vi "EnFlo_Tun_Heater_Control.vi"(1 "Heaters Enabled time (s)":dbl, 2 "Heaters Just Enabled":bool, 3 "Ch Names":string[](array[string]), 4 "Values":dbl[](array[numeric]) format="%.2f") -> ()   [LabVIEW 2016]
uses:
  ADAM Client/Sub VIs/ADAM Controls/Search_mode.ctl
  <vilib>/Analysis/baseanly.llb/Mean (DBL).vi
  ADAM_Global.vi
  <vilib>/Analysis/NI_AALBase.lvlib
  <vilib>/Analysis/NI_AALPro.lvlib
panel:
  out "Upper limit on Power":dbl
  in  "Proportional Error Deadband":dbl=0.03
  out "Read Values OK":bool
  out "History Out":dbl[](array[numeric])
  out "Current Temp":dbl
  out "Setpoint":dbl
  out "Error Range":dbl
  in  "Index To Display":i32
  out "Feedback Temperature":string
  in  "Minimum Power Change in %":dbl=0.08
  in  "Total History":i32=450
  out "Proportional Term":dbl format="%#.1f"
  out "Control Sum":dbl format="%#.1f"
  out "Differential Term":dbl format="%#.1f"
  in  "Derivative History":i32=60
  out "Integral Term":dbl format="%#.1f"
  # "This is the Max - Min error for the Total History"
  # "When running at\nSteady Cond"
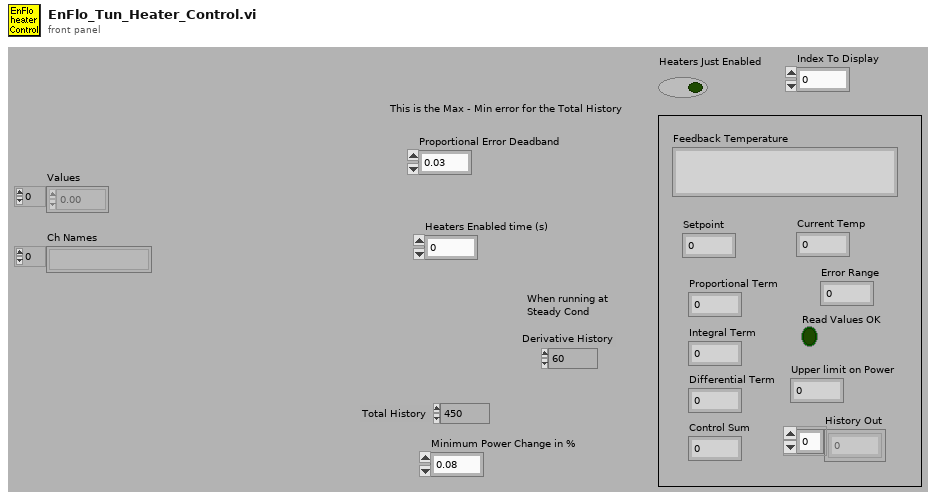
[diagram p1: front panel]
types:
  T1 = enum16{"On", "Off", "Always On", "Always Off", "Delete"}
  T2 = typedef "Search_mode.ctl" = enum16{"Between times", "All Times"}
  T3 = typedef "Ch_description_ADAM.ctl" = cluster{"Ch Name":string, "Type":T4, "Function":T5, "Ch State":T6, "Calibration type":T7, "A":dbl, "B":dbl, "C":dbl, "D":dbl, "Comments":string, "Address":T8, "String":string, "Duty":u16}
  T4 = typedef "Module_type_ADAM.ctl" = string
  T5 = typedef "Function_ADAM.ctl" = enum16{"Analogue Input", "Digital Input", "Event counter", "Event rate", "Analogue Output", "Digital Output", "Relay Output"}
  T6 = typedef "Channel_State.ctl" = enum16{"On", "Off", "Always On", "Always Off"}
  T7 = typedef "Calib_type_ADAM.ctl" = enum16{"Raw", "Bx + A", "Cx^2 + Bx + A", "Dx^3 + Cx^2 + Bx + A", "In Band", "Hi-Tec Q", "Hi-Tec M_dot", "Text"}
  T8 = typedef "Address.ctl" = cluster{"Main":i32, "Ch.":i32, "Sub":i32, "Port Name":string}
  T9 = cluster{"Centre Times":dbl[], "Output array":dbl[]}
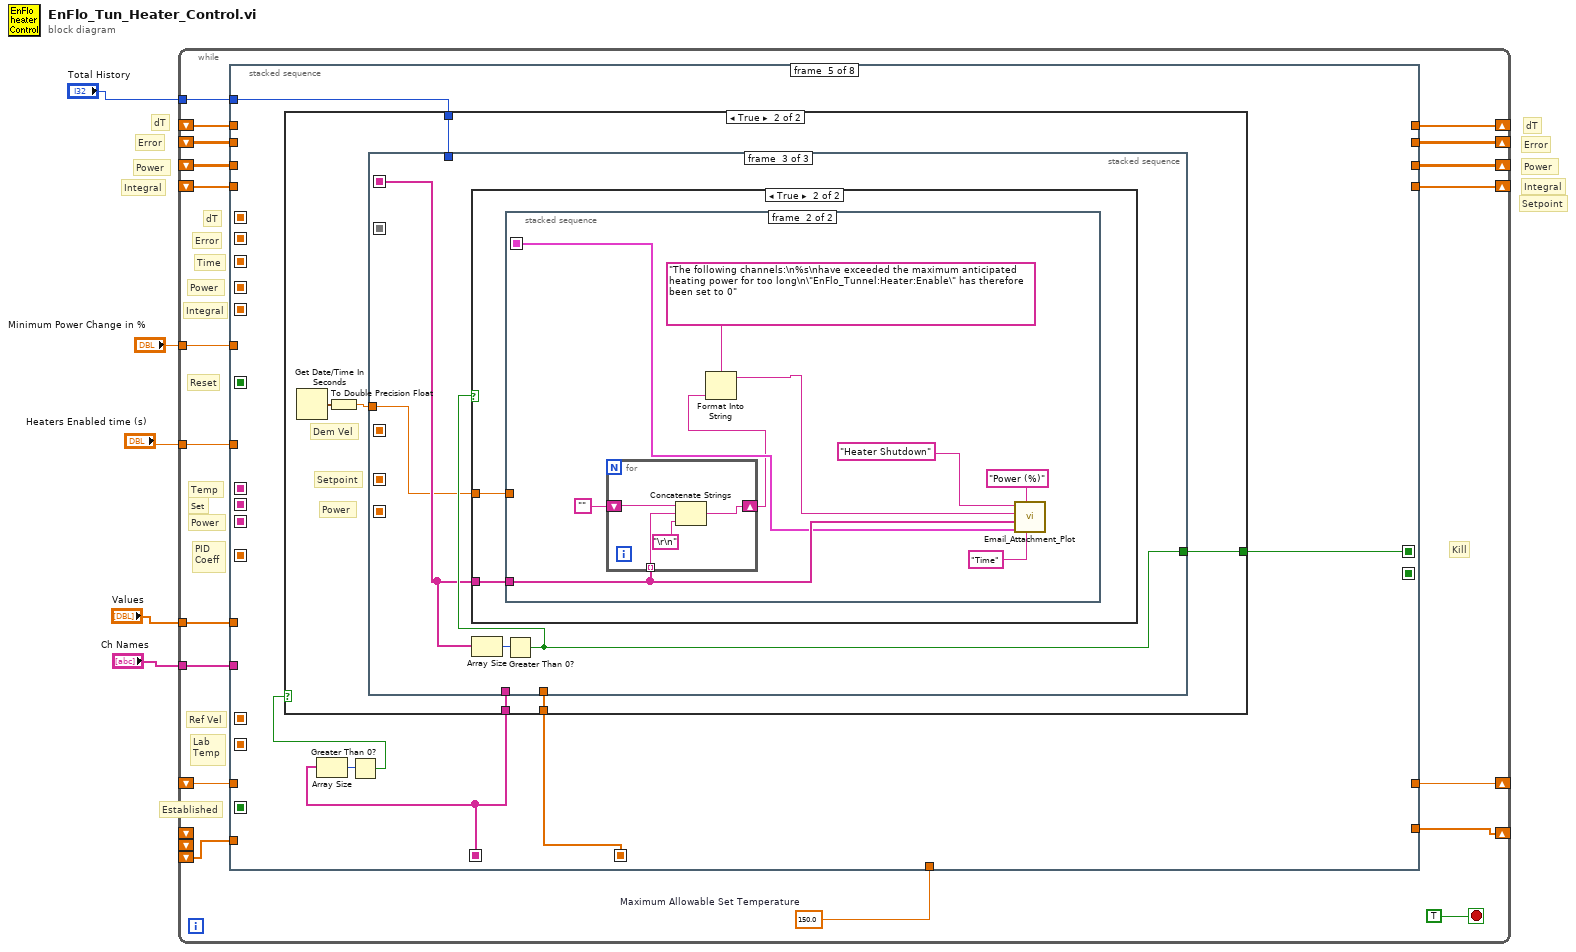
[diagram p0: block diagram]
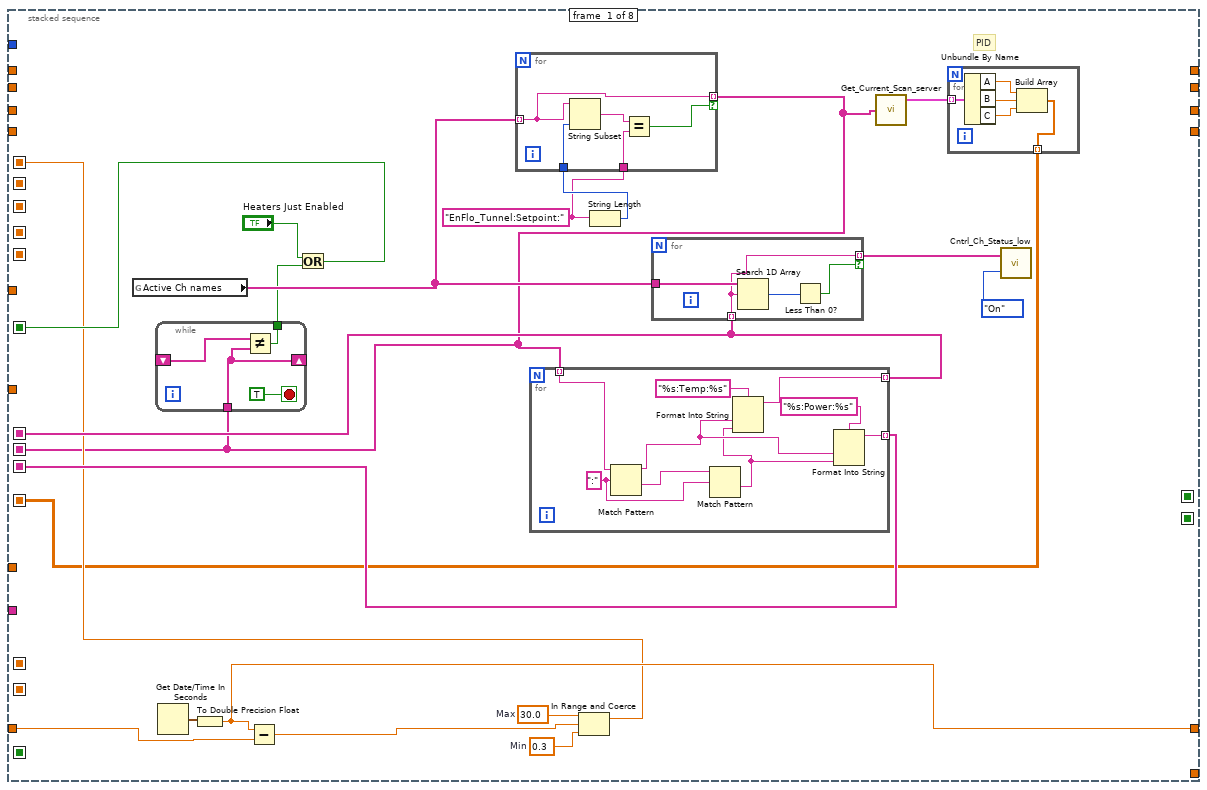
[diagram p2: hidden frame]
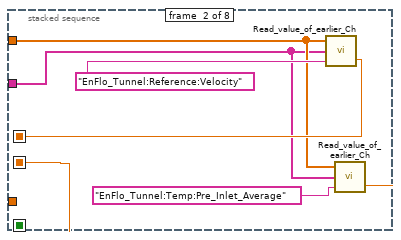
[diagram p3: hidden frame]
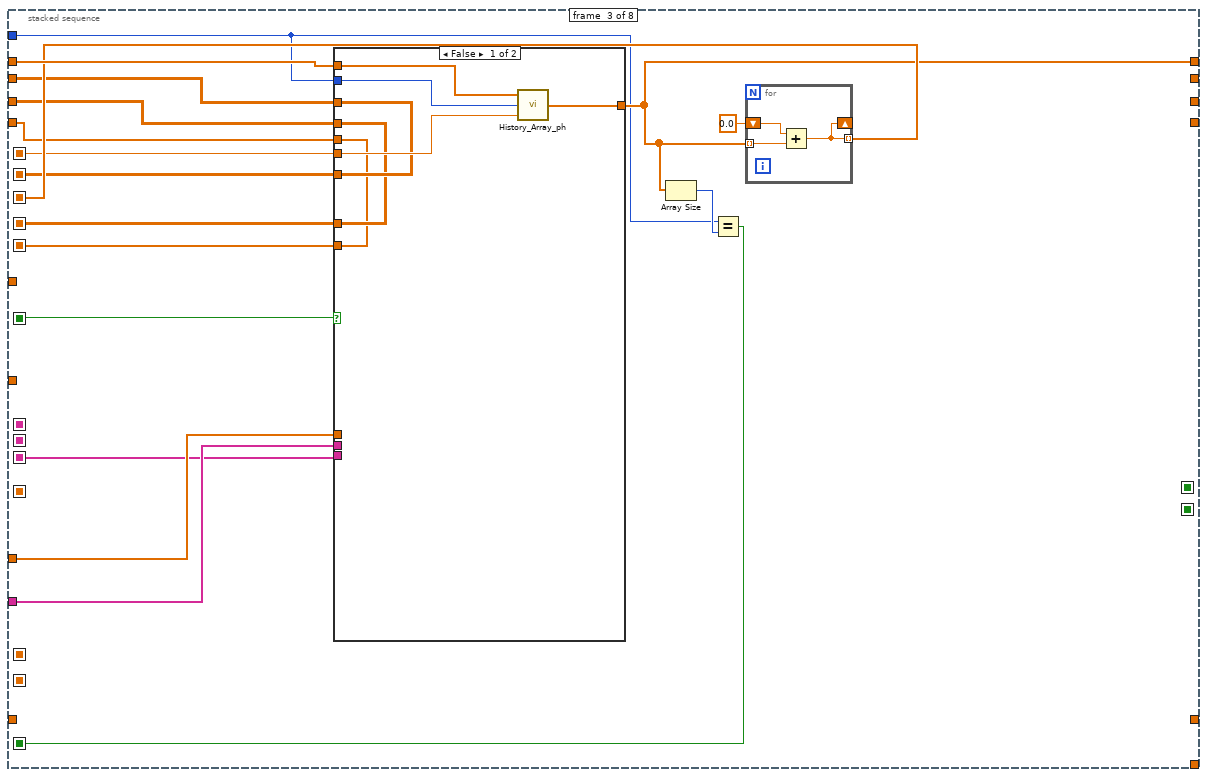
[diagram p4: hidden frame]
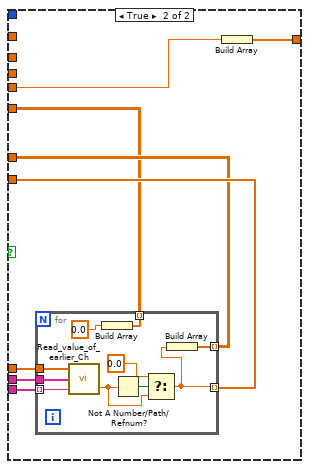
[diagram p5: hidden frame]
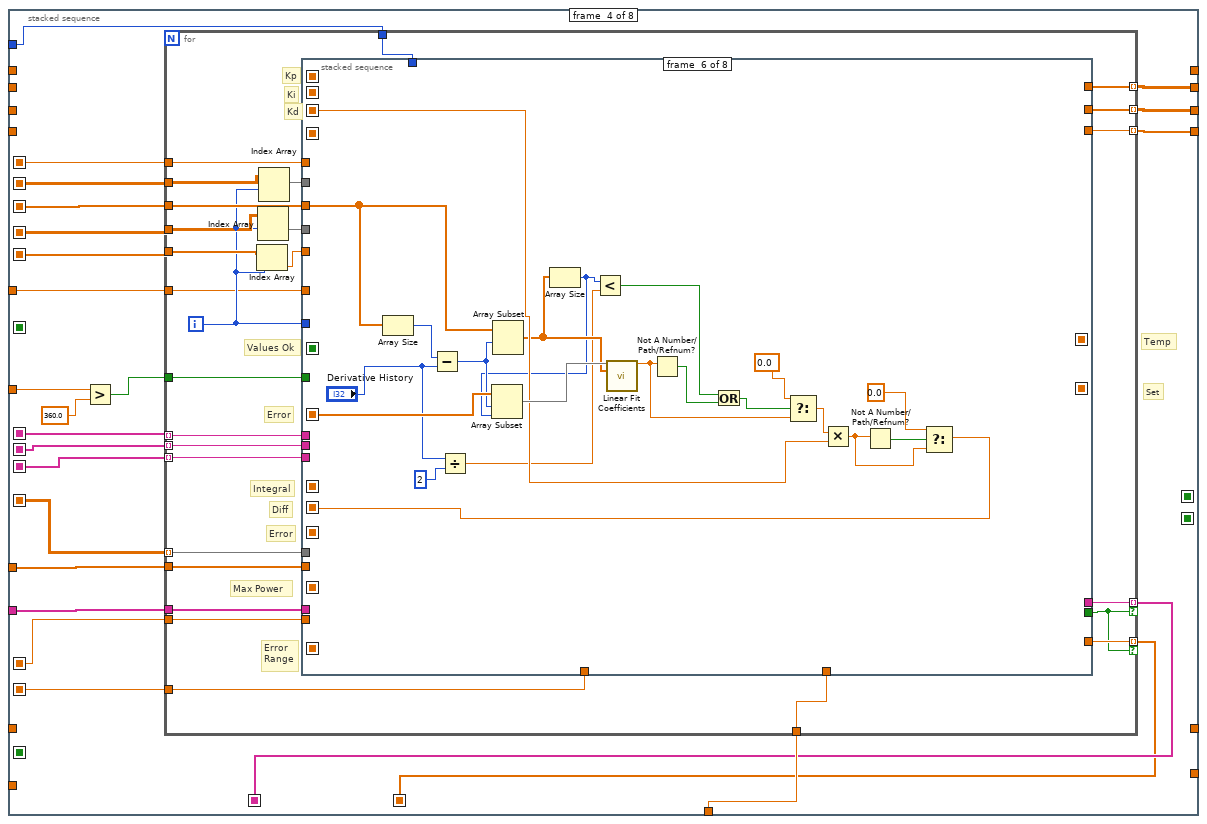
[diagram p6: hidden frame]
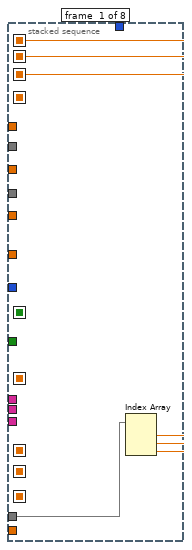
[diagram p7: hidden frame]
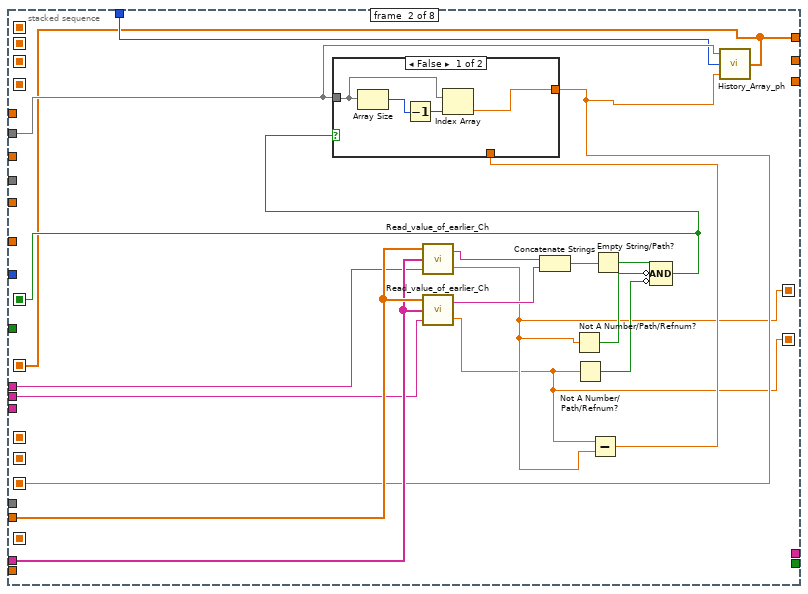
[diagram p8: hidden frame]
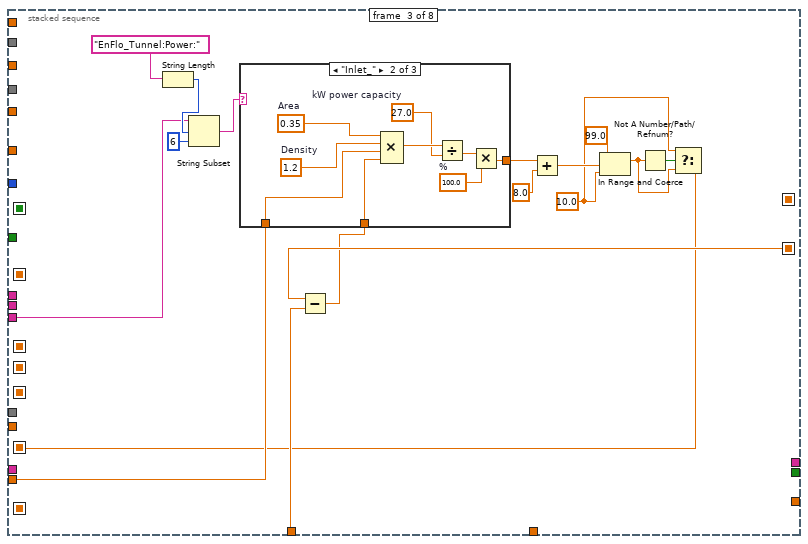
[diagram p10: hidden frame]
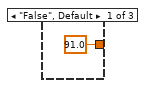
[diagram p11: hidden frame]
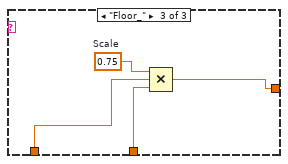
[diagram p12: hidden frame]
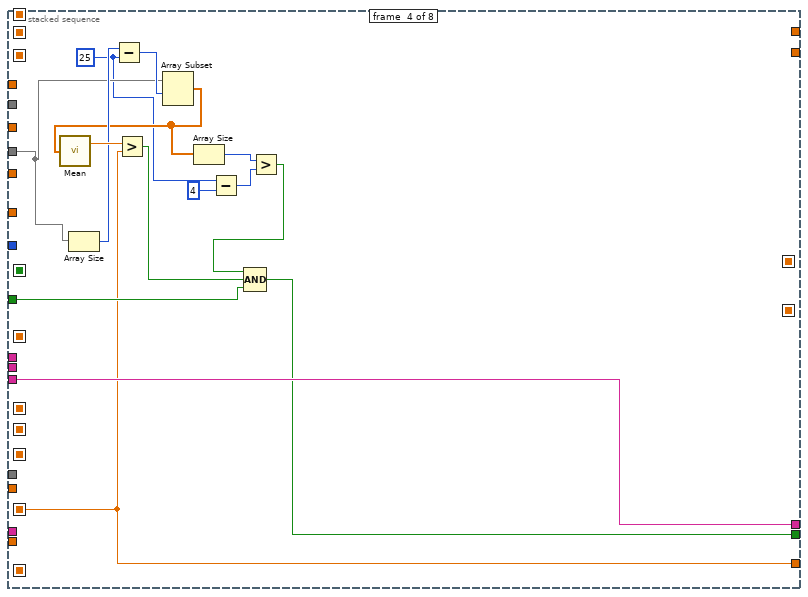
[diagram p13: hidden frame]
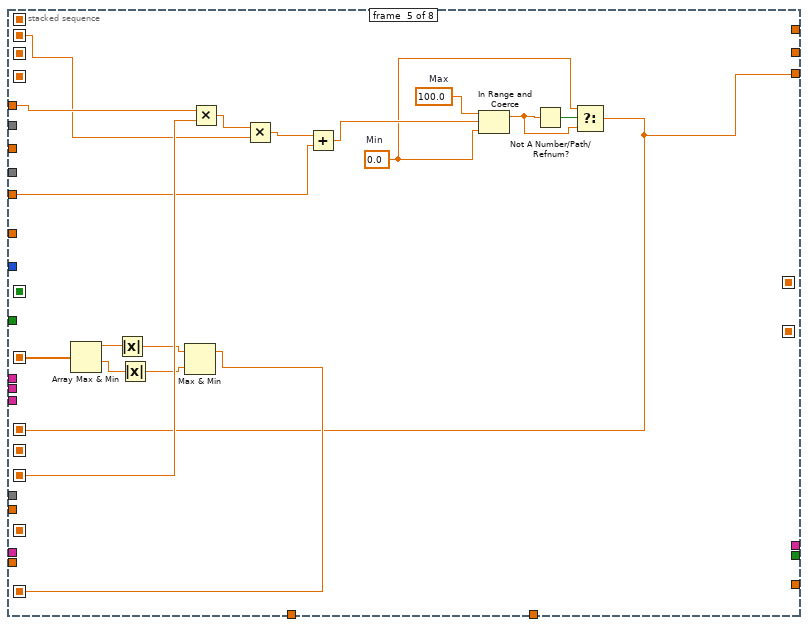
[diagram p14: hidden frame]
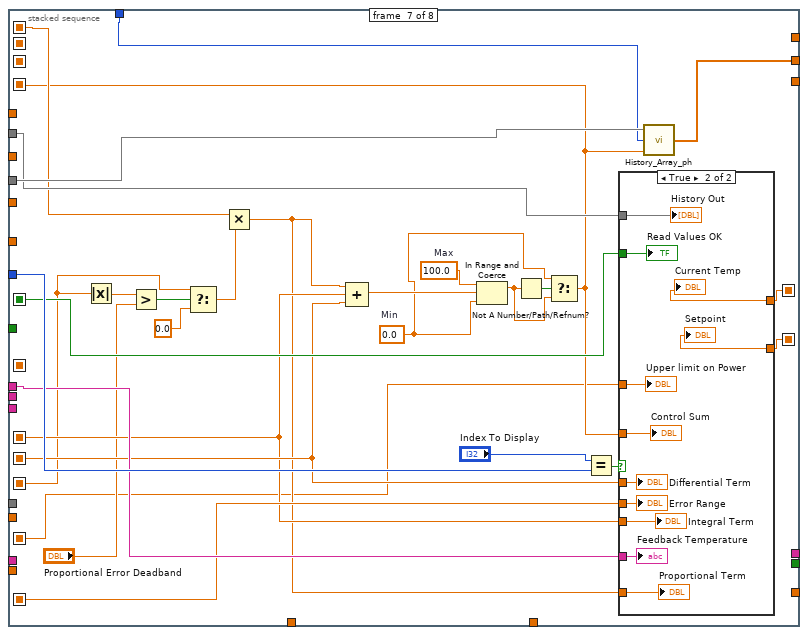
[diagram p15: hidden frame]
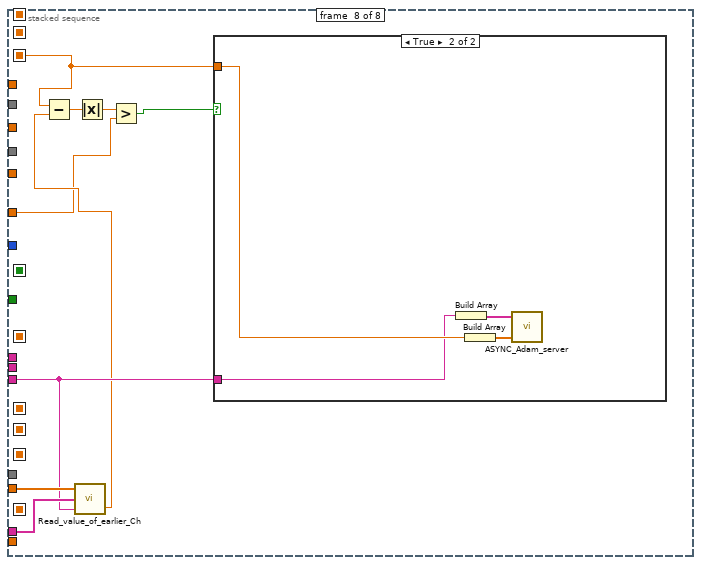
[diagram p17: hidden frame]
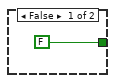
[diagram p19: hidden frame]
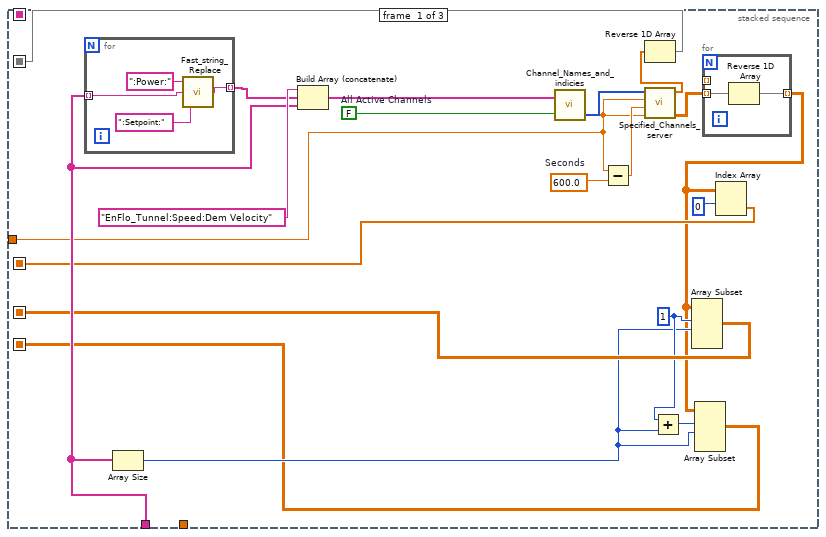
[diagram p20: hidden frame]
diagram:
  # "Integral"
  # "Power"
  # "Error"
  # "dT"
  # "Setpoint"
  # "Power"
  # "Integral"
  # "Error"
  # "dT"
  n1 = while {
    shift-right: [w22] -> _
    shift-left: _ -> [w23]
    shift-right: [w18] -> _
    shift-left: _ -> [w21]
    shift-right: [w20] -> _
    shift-left: _ -> [w19]
    shift-right: [w16] -> _
    shift-left: _ -> [w17]
    shift-right: [w14] -> _
    shift-left: _ -> [w15]
    tunnel: "Total History" -> [w13]
    tunnel: "Ch Names" -> [w11]
    tunnel: "Values" -> [w10]
    tunnel: "Minimum Power Change in %" -> [w9]
    shift-right: [w8] -> _
    shift-left: _ -> [_]
    shift-left: _ -> [_]
    shift-left: _ -> [w7]
    tunnel: "Heaters Enabled time (s)" -> [w6]
    stop <- TRUE stop-if-true
    w12 = 150.0  # Maximum Allowable Set Temperature
    # "Lab\nTemp"
    # "Ref Vel"
    # "Established"
    # "PID\nCoeff"
    # "dT"
    # "Integral"
    # "Power"
    # "Error"
    # "Reset"
    # "Kill"
    # "Power"
    # "Set"
    # "Temp"
    # "Time"
    n2 = stacked-sequence {
      seq-local: [_ _ w92 _ _ _ _ _] -> [_ _ _ w146 _ _ _ _]
      seq-local: [w35 _ _ _ _ _ _ _] -> [_ _ _ w143 _ _ w509 _]
      seq-local: [w26 _ _ _ _ _ _ _] -> [_ _ _ w142 _ _ w508 _]
      seq-local: [w42 _ _ _ _ _ _ _] -> [_ _ w82 w141 _ _ w511 _]
      seq-local: [_ _ _ w125 _ _ _ _] -> [_ _ _ _ w343 _ _ _]
      seq-local: [_ _ _ _ w341 _ _ _] -> [_ _ _ _ _ w468 _ _]
      seq-local: [_ _ _ _ _ w469 _ _] -> [_ _ _ _ _ _ _ w571]
      seq-local: [w29 _ _ _ _ _ _ _] -> [_ _ w91 w136 _ _ _ _]
      seq-local: [w30 _ _ _ _ _ _ _] -> [_ _ w94 _ _ _ _ _]
      seq-local: [_ _ w90 _ _ _ _ _] -> [_ _ _ w133 _ _ _ _]
      seq-local: [_ _ w88 _ _ _ _ _] -> [_ _ _ w134 _ _ _ _]
      seq-local: [_ _ w86 _ _ _ _ _] -> [_ _ _ w135 _ _ _ _]
      seq-local: [w27 _ _ _ _ _ _ _] -> [_ _ _ w131 _ _ _ _]
      seq-local: [_ _ w78 _ _ _ _ _] -> [_ _ _ _ _ _ w500 _]
      seq-local: [_ w76 _ _ _ _ _ _] -> [_ _ _ w127 _ _ _ _]
      seq-local: [_ w72 _ _ _ _ _ _] -> [_ _ _ w126 _ _ _ _]
      seq-local: [_ _ _ w124 _ _ _ _] -> [_ _ _ _ w340 _ _ _]
      tunnel: w23 -> [_ _ w95 _ _ _ _ _]
      tunnel: [_ _ w81 _ _ _ _ _] -> w22
      tunnel: w21 -> [_ _ w89 _ _ _ _ _]
      tunnel: [w36 _ _ _ _ _ _ _] -> w20
      tunnel: w19 -> [w38 _ _ _ _ _ _ _]
      tunnel: [_ _ _ w147 _ _ _ _] -> w18
      tunnel: w17 -> [_ _ w87 _ _ _ w510 _]
      tunnel: [_ _ _ w145 _ _ _ _] -> w16
      tunnel: w15 -> [_ _ w85 _ _ _ _ _]
      tunnel: [_ _ _ w144 _ _ _ _] -> w14
      tunnel: w13 -> [_ _ w79 w137 w344 w470 _ _]
      tunnel: w12 -> [_ _ _ w140 _ w462 _ _]
      tunnel: w11 -> [_ w74 w83 w139 _ w465 w506 _]
      tunnel: w10 -> [_ w75 w84 w138 _ w464 w507 _]
      tunnel: w9 -> [_ _ _ w132 _ _ w503 _]
      tunnel: [_ _ _ _ _ _ w496 _] -> w8
      tunnel: w7 -> [_ _ _ _ _ _ w495 _]
      tunnel: w6 -> [_ _ _ w130 _ _ _ _]
      frame #0 {
        w40 = 0.3  # Min
        w39 = 30.0  # Max
        w43 = "EnFlo_Tunnel:Setpoint:"
        # "PID"
        n3 = global read "ADAM_Global.vi" "Active Ch names"() -> (w33:string[])
        n4 = Get Date/Time In Seconds() -> (seconds since 1Jan1904=w41:timestamp)
        n5 = To Double Precision Float(number=w41) -> (double precision float=w36:dbl)
        n6 = Subtract(x=w36, y=w38) -> (x-y=w37:dbl)
        n7 = In Range and Coerce(upper limit=w39, x=w37, lower limit=w40) -> (coerced(x)=w29:dbl)  [unwired: 1 out]
        n8 = String Length(string=w43) -> (length=w44:i32)
        n9 = for {
          tunnel: w33 -> [w59] mode=indexing
          tunnel: w44 -> [w62]
          tunnel: w43 -> [w61]
          tunnel: [w59] -> w26 mode=indexing if=w58
          n10 = String Subset(string=w59, length (rest)=w62) -> (substring=w60:string)  [unwired: 1 out]
          n11 = Equal?(x=w60, y=w61) -> (x = y?=w58:bool)
        }
        n12 = while {
          shift-right: [w53] -> _
          shift-left: _ -> [w52]
          tunnel: w26 -> [w53]
          tunnel: [w51] -> w31
          stop <- TRUE stop-if-true
          n13 = Not Equal?(x=w52, y=w53) -> (x != y?=w51:bool)
        }
        n14 = Or(x="Heaters Just Enabled", y=w31) -> (x .or. y?=w30:bool)
        n15 = for {
          tunnel: w26 -> [w63] mode=indexing
          tunnel: [w64] -> w42 mode=indexing
          tunnel: [w65] -> w35 mode=indexing
          w70 = ":" ("regular expression")
          n16 = Match Pattern(string=w63, regular expression=w70) -> (before substring=w67:string, after substring=w71:string)  [unwired: 3 out]
          n17 = Match Pattern(string=w71, regular expression=w70) -> (after substring=w66:string)  [unwired: 4 out]
          n18 = Format Into String(format string="%s:Temp:%s", w67, w66) -> (resulting string=w65:string)  [unwired: 2 in, 1 out]
          n19 = Format Into String(format string="%s:Power:%s", w67, w66) -> (resulting string=w64:string)  [unwired: 2 in, 1 out]
        }
        n20 = for {
          tunnel: w35 -> [w56] mode=indexing
          tunnel: w33 -> [w57]
          tunnel: [w56] -> w25 mode=indexing if=w54
          n21 = Search 1D Array(1D array=w57, element=w56) -> (index of element=w55:i32)  [unwired: 1 in]
          n22 = Less Than 0?(x=w55) -> (x < 0?=w54:bool)
        }
        n23 = call "Get_Current_Scan_server.vi"("Desired Channels"=w26) -> ("Ch Description Array"=w28:T3[])  [unwired: 2 out]
        n24 = for {
          tunnel: w28 -> [w49] mode=indexing
          tunnel: [w45] -> w27 mode=indexing
          n25 = Unbundle By Name(w49) -> ("A"=w48:dbl, "B"=w47:dbl, "C"=w46:dbl)
          n26 = Build Array(w48, w47, w46) -> (w45:dbl[])
        }
        n27 = call "Cntrl_Ch_Status_low.vi"("Mode"=T1."On", "Channel names"=w25) -> ()  [unwired: 1 out]
      }
      frame #1 {
        n28 = call "Read_value_of_earlier_Ch.vi"("Desired Ch to Read"="EnFlo_Tunnel:Reference:Velocity", "Ch names"=w74, "Present scan array"=w75) -> ("Value"=w76:dbl)  [unwired: 1 in, 1 out]
        n29 = call "Read_value_of_earlier_Ch.vi"("Desired Ch to Read"="EnFlo_Tunnel:Temp:Pre_Inlet_Average", "Ch names"=w74, "Present scan array"=w75) -> ("Value"=w72:dbl)  [unwired: 1 in, 1 out]
      }
      frame #2 {
        n30 = case shown="False" w94 {
          tunnel: [w105 w113] -> w81
          tunnel: w95 -> [w104 _]
          tunnel: w79 -> [w103 _]
          tunnel: w91 -> [w102 w112]
          tunnel: [w101 w106] -> w90
          tunnel: w89 -> [w101 _]
          tunnel: [w100 w107] -> w88
          tunnel: w87 -> [w100 _]
          tunnel: [w99 w108] -> w86
          tunnel: w85 -> [w99 _]
          tunnel: w84 -> [_ w111]
          tunnel: w83 -> [_ w110]
          tunnel: w82 -> [_ w109]
          frame False {
            n31 = call "History_Array_ph.vi"("Current Value"=w102, "Desired Length"=w103, "History In"=w104) -> ("History Out"=w105:dbl[])
          }
          frame True {
            n32 = for {
              tunnel: w111 -> [w123]
              tunnel: w110 -> [w122]
              tunnel: w109 -> [w121] mode=indexing
              tunnel: [w114] -> w108 mode=indexing
              tunnel: [w120] -> w107 mode=indexing
              tunnel: [w118] -> w106 mode=indexing
              n33 = call "Read_value_of_earlier_Ch.vi"("Desired Ch to Read"=w121, "Ch names"=w122, "Present scan array"=w123) -> ("Value"=w116:dbl)  [unwired: 1 in, 1 out]
              n34 = Build Array(0.0) -> (w118:dbl[])
              n35 = Not A Number/Path/Refnum?(number/path/refnum=w116) -> (NaN/Path/Refnum?=w117:bool)
              n36 = Select(t=0.0, s=w117, f=w116) -> (s? t:f=w114:dbl)
              n37 = Build Array(w114) -> (w120:dbl[])
            }
            n38 = Build Array(w112) -> (w113:dbl[])
          }
        }
        n39 = Array Size(array=w81) -> (size(s)=w80:i32)
        n40 = Equal?(x=w79, y=w80) -> (x = y?=w78:bool)
        n41 = for {
          shift-right: [w97] -> _
          shift-left: 0.0 ("element") -> [w98]
          tunnel: [w97] -> w92 mode=indexing
          tunnel: w81 -> [w96] mode=indexing
          n42 = Add(x=w98, y=w96) -> (x+y=w97:dbl)
        }
      }
      frame #3 {
        # "Temp"
        # "Set"
        n43 = Greater?(x=w130, y=360.0) -> (0:w128:bool)
        n44 = for {
          tunnel: w138 -> [w161]
          tunnel: w139 -> [w160]
          tunnel: [w174] -> w147 mode=indexing
          tunnel: w133 -> [w164]
          tunnel: w136 -> [w173]
          tunnel: w146 -> [w166]
          tunnel: [w172] -> w145 mode=indexing
          tunnel: w134 -> [w165]
          tunnel: [w171] -> w144 mode=indexing
          tunnel: w135 -> [w167]
          tunnel: w143 -> [w170] mode=indexing
          tunnel: w142 -> [w159] mode=indexing
          tunnel: w141 -> [w169] mode=indexing
          tunnel: w140 -> [w168]
          tunnel: w137 -> [w163]
          tunnel: w132 -> [w155]
          tunnel: w131 -> [w154] mode=indexing
          tunnel: w128 -> [w153]
          tunnel: w127 -> [w152]
          tunnel: w126 -> [w151]
          tunnel: [w150] -> w125 mode=indexing if=w148
          tunnel: [w149] -> w124 mode=indexing if=w148
          i -> [w162]
          # "Max Power"
          # "Kd"
          # "Ki"
          # "Kp"
          # "Values Ok"
          # "Error\nRange"
          # "Integral"
          # "Error"
          # "Error"
          # "Diff"
          n45 = Index Array(array=w167, index=w162) -> (element=w158:dbl)
          n46 = Index Array(array=w165, index (row)=w162) -> (element=w156:dbl[])  [unwired: 1 in]
          n47 = Index Array(array=w164, index (row)=w162) -> (element=w157:dbl[])  [unwired: 1 in]
          n48 = stacked-sequence {
            seq-local: [_ _ _ _ _ w282 _ _] -> [_ _ _ _ _ _ w301 _]
            seq-local: [_ w182 _ _ _ _ _ _] -> [_ _ _ _ w265 _ w296 _]
            seq-local: [_ w181 _ _ _ _ _ _] -> [_ _ _ _ w263 w279 _ _]
            seq-local: [_ _ _ _ w249 _ _ _] -> [_ _ _ _ _ _ w300 _]
            seq-local: [_ _ _ _ _ _ w289 _] -> [_ _ _ _ _ _ _ w332]
            seq-local: [_ w183 _ _ _ _ _ _] -> [_ _ _ _ _ _ w302 _]
            seq-local: [_ _ _ _ w254 _ _ _] -> [_ _ _ _ _ _ w306 _]
            seq-local: [_ w180 _ _ _ _ _ _] -> [_ _ _ _ _ _ w304 _]
            seq-local: [_ w179 _ _ _ _ _ _] -> [_ _ w209 _ _ _ w305 _]
            seq-local: [w177 _ _ _ _ _ _ _] -> [_ _ _ _ _ _ w292 _]
            seq-local: [w176 _ _ _ _ _ _ _] -> [_ _ _ _ w252 _ _ _]
            seq-local: [w175 _ _ _ _ _ _ _] -> [_ _ _ _ _ w276 _ _]
            seq-local: [_ _ w203 _ _ _ _ _] -> [_ _ _ w233 _ _ w287 _]
            tunnel: w161 -> [_ w196 _ _ _ _ _ w335]
            tunnel: w160 -> [_ w195 _ _ _ _ _ w334]
            tunnel: [_ w181 _ _ _ _ _ _] -> w174
            tunnel: w157 -> [_ w185 _ _ _ _ w303 _]
            tunnel: w173 -> [_ _ _ _ w253 _ _ _]
            tunnel: w166 -> [_ _ _ _ _ w275 _ _]
            tunnel: [_ _ _ _ _ _ w313 _] -> w172
            tunnel: w156 -> [_ _ _ w244 _ _ w312 _]
            tunnel: [_ _ _ _ w249 _ _ _] -> w171
            tunnel: w158 -> [_ _ _ _ w264 _ _ _]
            tunnel: w170 -> [_ w186 _ _ _ _ w307 _]
            tunnel: w159 -> [_ w187 _ _ _ _ _ _]
            tunnel: w169 -> [_ _ w210 w235 _ _ _ w333]
            tunnel: w168 -> [_ _ _ _ _ _ _ _]
            tunnel: w163 -> [_ w184 _ _ _ _ w311 _]
            tunnel: w162 -> [_ _ _ _ _ _ w309 _]
            tunnel: w155 -> [_ _ _ _ _ _ _ w327]
            tunnel: w154 -> [w178 _ _ _ _ _ _ _]
            tunnel: w153 -> [_ _ _ w236 _ _ _ _]
            tunnel: w152 -> [_ _ w206 _ _ _ _ _]
            tunnel: w151 -> [_ _ w208 _ _ _ _ _]
            tunnel: [_ _ _ w235 _ _ _ _] -> w150
            tunnel: [_ _ _ w234 _ _ _ _] -> w148
            tunnel: [_ _ _ w233 _ _ _ _] -> w149
            frame #0 {
              n49 = Index Array(array=w178) -> (element #1=w177:dbl, element #2=w176:dbl, element #3=w175:dbl)  [unwired: 3 in]
            }
            frame #1 {
              n50 = call "Read_value_of_earlier_Ch.vi"("Desired Ch to Read"=w186, "Ch names"=w195, "Present scan array"=w196) -> ("Value"=w180:dbl, "Scan comment"=w194:string)  [unwired: 1 in]
              n51 = call "Read_value_of_earlier_Ch.vi"("Desired Ch to Read"=w187, "Ch names"=w195, "Present scan array"=w196) -> ("Value"=w179:dbl, "Scan comment"=w193:string)  [unwired: 1 in]
              n52 = Concatenate Strings(w194, w193) -> (w192:string)
              n53 = Not A Number/Path/Refnum?(number/path/refnum=w180) -> (NaN/Path/Refnum?=w190:bool)
              n54 = Not A Number/Path/Refnum?(number/path/refnum=w179) -> (NaN/Path/Refnum?=w189:bool)
              n55 = Subtract(x=w179, y=w180) -> (x-y=w188:dbl)
              n56 = Empty String/Path?(string/path=w192) -> (empty?=w191:bool)
              n57 = Compound Arithmetic op=AND(w191, invert w190, invert w189) -> (w183:bool)
              n58 = case shown="False" w183 {
                tunnel: w185 -> [w197 _]
                tunnel: [w200 w201] -> w182
                tunnel: w188 -> [_ w201]
                frame False {
                  n59 = Array Size(array=w197) -> (size(s)=w198:i32)
                  n60 = Decrement(x=w198) -> (x-1=w199:i32)
                  n61 = Index Array(array=w197, index=w199) -> (element=w200:dbl)
                }
                frame True {
                }
              }
              n62 = call "History_Array_ph.vi"("Current Value"=w182, "Desired Length"=w184, "History In"=w185) -> ("History Out"=w181:dbl[])
            }
            frame #2 {
              w202 = 10.0 ("lower limit")
              n63 = String Length(string="EnFlo_Tunnel:Power:") -> (length=w217:i32)
              n64 = String Subset(string=w210, offset (0)=w217, length (rest)=6 ("length (rest)")) -> (substring=w215:string)
              n65 = Subtract(x=w209, y=w208) -> (x-y=w207:dbl)
              n66 = case shown="\"Inlet_\"" w215 {
                tunnel: w206 -> [_ w226 w232]
                tunnel: w207 -> [_ w225 w231]
                tunnel: [91.0 w220 w230] -> w214
                frame "False", Default {
                }
                frame "Inlet_" {
                  w221 = 100.0  # %
                  w223 = 27.0  # kW power capacity
                  w227 = 1.2  # Density
                  w228 = 0.35  # Area
                  n67 = Compound Arithmetic op=MULTIPLY(w228, w227, w226, w225) -> (w224:dbl)
                  n68 = Divide(x=w224, y=w223) -> (x/y=w222:dbl)
                  n69 = Multiply(x=w222, y=w221) -> (x*y=w220:dbl)
                }
                frame "Floor_" {
                  w229 = 0.75  # Scale
                  n70 = Compound Arithmetic op=MULTIPLY(w229, w232, w231) -> (w230:dbl)
                }
              }
              n71 = Add(x=w214, y=8.0) -> (x+y=w212:dbl)
              n72 = In Range and Coerce(upper limit=99.0, x=w212, lower limit=w202) -> (coerced(x)=w204:dbl)  [unwired: 1 out]
              n73 = Not A Number/Path/Refnum?(number/path/refnum=w204) -> (NaN/Path/Refnum?=w205:bool)
              n74 = Select(t=w202, s=w205, f=w204) -> (s? t:f=w203:dbl)
            }
            frame #3 {
              w241 = 25 ("y")
              n75 = Array Size(array=w244) -> (size(s)=w246:i32)
              n76 = Subtract(x=w246, y=w241) -> (x-y=w245:i32)
              n77 = Array Subset(array=w244, index=w245) -> (w243:dbl[])  [unwired: 1 in]
              n78 = call-poly <vilib>:"Mean.vi"("X"=w243) -> ("mean"=w247:dbl)  [unwired: 1 out]
              n79 = Greater?(x=w247, y=w233) -> (0:w238:bool)
              n80 = Array Size(array=w243) -> (size(s)=w242:i32)
              n81 = Subtract(x=w241, y=4) -> (x-y=w239:i32)
              n82 = Greater?(x=w242, y=w239) -> (0:w237:bool)
              n83 = Compound Arithmetic op=AND(w237, w238, w236) -> (w234:bool)
            }
            frame #4 {
              w248 = 0.0  # Min
              w262 = 100.0  # Max
              n84 = Array Max & Min(array=w263) -> (max value=w258:dbl, min value=w257:dbl)  [unwired: 2 out]
              n85 = Absolute Value(x=w258) -> (abs(x)=w255:dbl)
              n86 = Absolute Value(x=w257) -> (abs(x)=w256:dbl)
              n87 = Max & Min(x=w255, y=w256) -> (max(x,y)=w254:dbl)  [unwired: 1 out]
              n88 = Multiply(x=w253, y=w265) -> (x*y=w261:dbl)
              n89 = Multiply(x=w261, y=w252) -> (x*y=w260:dbl)
              n90 = Add(x=w260, y=w264) -> (x+y=w259:dbl)
              n91 = In Range and Coerce(upper limit=w262, x=w259, lower limit=w248) -> (coerced(x)=w250:dbl)  [unwired: 1 out]
              n92 = Not A Number/Path/Refnum?(number/path/refnum=w250) -> (NaN/Path/Refnum?=w251:bool)
              n93 = Select(t=w248, s=w251, f=w250) -> (s? t:f=w249:dbl)
            }
            frame #5 {
              n94 = Array Size(array=w275) -> (size(s)=w274:i32)
              n95 = Subtract(x=w274, y="Derivative History") -> (x-y=w277:i32)
              n96 = Divide(x="Derivative History", y=2) -> (x/y=w270:dbl)
              n97 = Array Subset(array=w275, index=w277) -> (w273:dbl[])  [unwired: 1 in]
              n98 = Array Size(array=w273) -> (size(s)=w266:i32)
              n99 = Array Subset(array=w279, index=w277, length=w266) -> (w278:dbl[])
              n100 = Less?(x=w266, y=w270) -> (x < y?=w268:bool)
              n101 = call <vilib>:"Linear Fit Coefficients.vi"("Y"=w278, "X"=w273) -> ("slope"=w286:dbl)  [unwired: 3 in, 10 out]
              n102 = Not A Number/Path/Refnum?(number/path/refnum=w286) -> (NaN/Path/Refnum?=w269:bool)
              n103 = Or(x=w268, y=w269) -> (x .or. y?=w267:bool)
              n104 = Select(t=0.0 ("f"), s=w267, f=w286) -> (s? t:f=w284:dbl)
              n105 = Multiply(x=w284, y=w276) -> (x*y=w281:dbl)
              n106 = Not A Number/Path/Refnum?(number/path/refnum=w281) -> (NaN/Path/Refnum?=w283:bool)
              n107 = Select(t=0.0, s=w283, f=w281) -> (s? t:f=w282:dbl)
            }
            frame #6 {
              w288 = 0.0  # Min
              w315 = 100.0  # Max
              n108 = Absolute Value(x=w296) -> (abs(x)=w298:dbl)
              n109 = Greater?(x=w298, y="Proportional Error Deadband") -> (0:w297:bool)
              n110 = Select(t=w296, s=w297, f=0.0) -> (s? t:f=w295:dbl)
              n111 = Multiply(x=w292, y=w295) -> (x*y=w299:dbl)
              n112 = Compound Arithmetic op=ADD(w299, w300, w301) -> (w314:dbl)
              n113 = In Range and Coerce(upper limit=w315, x=w314, lower limit=w288) -> (coerced(x)=w290:dbl)  [unwired: 1 out]
              n114 = Not A Number/Path/Refnum?(number/path/refnum=w290) -> (NaN/Path/Refnum?=w291:bool)
              n115 = Select(t=w288, s=w291, f=w290) -> (s? t:f=w289:dbl)
              n116 = Equal?(x="Index To Display", y=w309) -> (x = y?=w308:bool)
              n117 = case shown="True" w308 {
                tunnel: w299 -> [_ w326]
                tunnel: w289 -> [_ w325]
                tunnel: w301 -> [_ w324]
                tunnel: w300 -> [_ w323]
                tunnel: w307 -> [_ w322]
                tunnel: w306 -> [_ w321]
                tunnel: w305 -> [_ w320]
                tunnel: w304 -> [_ w319]
                tunnel: w303 -> [_ w318]
                tunnel: w302 -> [_ w317]
                tunnel: w287 -> [_ w316]
                frame False {
                }
                frame True {
                  "Control Sum" <- w325
                  "Proportional Term" <- w326
                  "Differential Term" <- w324
                  "Integral Term" <- w323
                  "Feedback Temperature" <- w322
                  "Error Range" <- w321
                  "Setpoint" <- w320
                  "Current Temp" <- w319
                  "History Out" <- w318
                  "Read Values OK" <- w317
                  "Upper limit on Power" <- w316
                }
              }
              n118 = call "History_Array_ph.vi"("Current Value"=w289, "Desired Length"=w311, "History In"=w312) -> ("History Out"=w313:dbl[])
            }
            frame #7 {
              n119 = call "Read_value_of_earlier_Ch.vi"("Desired Ch to Read"=w333, "Ch names"=w334, "Present scan array"=w335) -> ("Value"=w331:dbl)  [unwired: 1 in, 1 out]
              n120 = Subtract(x=w332, y=w331) -> (x-y=w330:dbl)
              n121 = Absolute Value(x=w330) -> (abs(x)=w329:dbl)
              n122 = Greater?(x=w329, y=w327) -> (0:w328:bool)
              n123 = case shown="True" w328 {
                tunnel: w332 -> [_ w337]
                tunnel: w333 -> [_ w336]
                frame False {
                }
                frame True {
                  n124 = Build Array(w336) -> (w338:string[])
                  n125 = Build Array(w337) -> (w339:dbl[])
                  n126 = call "ASYNC_Adam_server.vi"("Values"=w339, "Channel Names"=w338) -> ()  [unwired: 1 in, 3 out]
                }
              }
            }
          }
        }
      }
      frame #4 {
        n127 = Array Size(array=w343) -> (size(s)=w345:i32)
        n128 = Greater Than 0?(x=w345) -> (x > 0?=w342:bool)
        n129 = case shown="True" w342 {
          tunnel: w344 -> [_ w351]
          tunnel: w343 -> [_ w352]
          tunnel: [FALSE w350] -> w341
          tunnel: w340 -> [_ w347]
          frame False {
          }
          frame True {
            # "Dem Vel"
            # "Power"
            # "Setpoint"
            n130 = Get Date/Time In Seconds() -> (seconds since 1Jan1904=w349:timestamp)
            n131 = To Double Precision Float(number=w349) -> (double precision float=w348:dbl)
            n132 = stacked-sequence {
              seq-local: [_ w380 _] -> [_ _ w428]
              seq-local: [w363 _ _] -> [_ w385 _]
              seq-local: [w359 _ _] -> [_ w386 _]
              seq-local: [w357 _ _] -> [_ w384 _]
              seq-local: [w354 _ _] -> [_ w383 _]
              tunnel: w352 -> [w365 w381 _]
              tunnel: w351 -> [_ _ _]
              tunnel: [_ _ w429] -> w350
              tunnel: w348 -> [w364 w382 w427]
              tunnel: w347 -> [_ w379 _]
              frame #0 {
                w362 = 1 ("index")
                w366 = 600.0  # Seconds
                w372 = FALSE  # All Active Channels
                n133 = for {
                  tunnel: w365 -> [w376] mode=indexing
                  tunnel: [w375] -> w367 mode=indexing
                  n134 = call "Fast_string_Replace.vi"("Replace match with:"=":Setpoint:" ("regular expression"), "Input String"=w376, "regular expression"=":Power:") -> ("Output String"=w375:string)  [unwired: 2 out]
                }
                n135 = Array Size(array=w365) -> (size(s)=w360:i32)
                n136 = Build Array (concatenate)("EnFlo_Tunnel:Speed:Dem Velocity", w367, w365) -> (w369:string[])
                n137 = call "Channel_Names_and_indicies.vi"("All Active Channels"=w372, "Desired Ch Names"=w369) -> ("Indicies"=w371:i32[])  [unwired: 1 out]
                n138 = Subtract(x=w364, y=w366) -> (x-y=w370:dbl)
                n139 = call "Specified_Channels_server.vi"("End time"=w364, "Start time"=w370, "Clients time"=w364, "Requested channels"=w371) -> ("Output array"=w356:dbl[][], "Centre Times"=w355:dbl[])  [unwired: 1 in, 3 out]
                n140 = Reverse 1D Array(array=w355) -> (reversed array=w354:dbl[])
                n141 = Add(x=w362, y=w360) -> (x+y=w361:i32)
                n142 = for {
                  tunnel: [w374] -> _ mode=indexing
                  tunnel: w356 -> [w374] mode=indexing
                  tunnel: [w373] -> w353 mode=indexing
                  n143 = Reverse 1D Array(array=w374) -> (reversed array=w373:dbl[])
                }
                n144 = Array Subset(array=w353, index (row)=w362, length (row)=w360) -> (w363:dbl[][])  [unwired: 2 in]
                n145 = Array Subset(array=w353, index (row)=w361, length (row)=w360) -> (w359:dbl[][])  [unwired: 2 in]
                n146 = Index Array(array=w353, index (row)=0) -> (element=w357:dbl[])  [unwired: 1 in]
              }
              frame #1 {
                n147 = for {
                  tunnel: w386 -> [w418] mode=indexing
                  tunnel: w385 -> [w416] mode=indexing
                  tunnel: w384 -> [w408]
                  tunnel: w383 -> [w398]
                  tunnel: w382 -> [w397]
                  tunnel: w381 -> [w389] mode=indexing
                  tunnel: [w389] -> w380 mode=indexing if=w388
                  tunnel: w379 -> [w387] mode=indexing
                  n148 = for {
                    tunnel: w418 -> [w426] mode=indexing
                    tunnel: [w424] -> w399
                    tunnel: w387 -> [w423]
                    i -> [w424]
                    stop <- w425 continue-if-true
                    n149 = Greater?(x=w426, y=w423) -> (0:w425:bool)
                  }
                  n150 = Index Array(array=w398, index=w399) -> (element=w396:dbl)
                  n151 = Add(x=10, y=w399) -> (x+y=w409:i32)
                  n152 = Subtract(x=w397, y=w396) -> (x-y=w395:dbl)
                  n153 = Array Subset(array=w416, length=w409) -> (w415:dbl[])  [unwired: 1 in]
                  n154 = Array Subset(array=w408, length=w409) -> (w410:dbl[])  [unwired: 1 in]
                  n155 = Array Max & Min(array=w415) -> (max value=w414:dbl, min value=w413:dbl)  [unwired: 2 out]
                  n156 = Array Max & Min(array=w410) -> (max value=w411:dbl, min value=w412:dbl)  [unwired: 2 out]
                  n157 = Match Pattern(string=w389, regular expression="ve_Side_") -> (offset past match=w393:i32)  [unwired: 1 in, 3 out]
                  n158 = Subtract(x=w414, y=w413) -> (x-y=w407:dbl)
                  n159 = Subtract(x=w411, y=w412) -> (x-y=w405:dbl)
                  n160 = Greater Or Equal To 0?(x=w393) -> (x >= 0?=w392:bool)
                  n161 = Multiply(x=w407, y=4.0) -> (x*y=w402:dbl)
                  n162 = Multiply(x=w405, y=100.0) -> (x*y=w403:dbl)
                  n163 = Max & Min(x=w403, y=w402) -> (max(x,y)=w401:dbl)  [unwired: 1 out]
                  n164 = Add(x=100.0, y=w401) -> (x+y=w391:dbl)
                  n165 = case shown="False" w392 {
                    tunnel: w391 -> [w419 w421]
                    tunnel: [w419 w420] -> w390
                    frame False {
                    }
                    frame True {
                      n166 = Multiply(x=w421, y=3.0) -> (x*y=w420:dbl)
                    }
                  }
                  n167 = Greater?(x=w395, y=w390) -> (0:w388:bool)
                }
              }
              frame #2 {
                n168 = Array Size(array=w428) -> (size(s)=w430:i32)
                n169 = Greater Than 0?(x=w430) -> (x > 0?=w429:bool)
                n170 = case shown="True" w429 {
                  tunnel: w428 -> [_ w432]
                  tunnel: w427 -> [_ w431]
                  frame False {
                  }
                  frame True {
                    n171 = stacked-sequence {
                      seq-local: [w434 _] -> [_ w449]
                      tunnel: w432 -> [w439 w451]
                      tunnel: w431 -> [w438 _]
                      frame #0 {
                        w433 = TRUE  # Contact All clients?
                        n172 = Subtract(x=w438, y=3000.0) -> (x-y=w436:dbl)
                        n173 = call "Channel_Names_and_indicies.vi"("All Active Channels"=FALSE, "Desired Ch Names"=w439) -> ("Indicies"=w442:i32[])  [unwired: 1 out]
                        n174 = call "Specified_Channels_server.vi"("Mode"=Search_mode."Between times", "End time"=w438, "Start time"=w436, "Clients time"=w438, "Requested channels"=w442) -> ("Output array"=w435:dbl[][], "Centre Times"=w443:dbl[])  [unwired: 3 out]
                        n175 = for {
                          tunnel: w443 -> [w446]
                          tunnel: w435 -> [w445] mode=indexing
                          tunnel: [w444] -> w434 mode=indexing
                          n176 = Bundle("Centre Times"=w446, "Output array"=w445) -> (w444:T9)  [unwired: 1 out]
                        }
                        n177 = call "Client_email_addresses.vi"("Contact All clients?"=w433) -> ()  [unwired: 2 in]
                      }
                      frame #1 {
                        n178 = for {
                          shift-right: [w456] -> w447
                          shift-left: "" -> [w459]
                          tunnel: w451 -> [w457] mode=indexing
                          n179 = Concatenate Strings(w459, w457, "\r\n") -> (w456:string)
                        }
                        n180 = Format Into String(format string="The following channels:\n%s\nhave exceeded the maximum anticipated heating power for too long\n\"EnFlo_Tunnel:Heater:Enable\" has therefore been set to 0", w447) -> (resulting string=w452:string)  [unwired: 2 in, 1 out]
                        n181 = call "Email_Attachment_Plot.vi"("X axis name"="Time", "Y axis name"="Power (%)", "XY Graph"=w449, "Series Names"=w451, "message"=w452, "subject ([No Subject])"="Heater Shutdown" ("t")) -> ()  [unwired: 1 out]
                      }
                    }
                  }
                }
              }
            }
          }
        }
      }
      frame #5 {
        w466 = "EnFlo_Tunnel:Temp:"
        n182 = String Length(string=w466) -> (length=w467:i32)
        n183 = for {
          shift-right: [w476] -> w460
          shift-left: "" -> [w477]
          tunnel: w465 -> [w480] mode=indexing
          tunnel: w467 -> [w481]
          tunnel: w466 -> [w478]
          tunnel: w464 -> [w475] mode=indexing
          tunnel: w462 -> [w474]
          n184 = String Subset(string=w480, length (rest)=w481) -> (substring=w479:string)  [unwired: 1 out]
          n185 = Equal?(x=w479, y=w478) -> (x = y?=w471:bool)
          n186 = Greater?(x=w475, y=w474) -> (0:w472:bool)
          n187 = And(x=w471, y=w472) -> (x .and. y?=w473:bool)
          n188 = case shown="True" w473 {
            tunnel: w480 -> [_ w483]
            tunnel: w477 -> [w482 w485]
            tunnel: [w482 w484] -> w476
            frame False {
            }
            frame True {
              n189 = Concatenate Strings(w485, w483, "\r\n") -> (w484:string)
            }
          }
        }
        n190 = Empty String/Path?(string/path=w460) -> (empty?=w461:bool)
        n191 = case shown="False" w461 {
          tunnel: w470 -> [_ _]
          tunnel: w462 -> [w488 _]
          tunnel: [TRUE w494] -> w469
          tunnel: w468 -> [_ w494]
          tunnel: w460 -> [w487 _]
          frame False {
            n192 = Format Into String(format string="The following channels have reached a temperature of  %d deg C\n\n%s\n\n\"EnFlo_Tunnel:Heater:Enable\" has therefore been set to 0", w488, w487) -> (resulting string=w490:string)  [unwired: 2 in, 1 out]
            n193 = call "Server_Emails.vi"("Client Name Contains"="EnFlo_Tunnel", "Message"=w490, "Subject"="Heater Shutdown" ("t")) -> ()  [unwired: 2 in, 3 out]
          }
          frame True {
          }
        }
      }
      frame #6 {
        w504 = ""
        # "Integer Precision on measure temp\nso that not too many emails are sent"
        n194 = Add(x=w503, y=0.2) -> (x+y=w501:dbl)
        n195 = for {
          tunnel: w511 -> [w541] mode=indexing
          tunnel: w510 -> [w545] mode=indexing
          shift-right: [w542] -> w505
          shift-left: w504 -> [w543]
          tunnel: w509 -> [w540] mode=indexing
          tunnel: w508 -> [w534] mode=indexing
          tunnel: w507 -> [w536]
          tunnel: w506 -> [w535]
          shift-right: [w538] -> w499
          shift-left: w504 -> [w539]
          tunnel: w501 -> [w537]
          tunnel: [w526] -> w496 mode=indexing
          tunnel: w495 -> [w528]
          i -> [w529]
          n196 = Index Array(array=w528, index=w529) -> (element=w525:dbl)
          n197 = call-poly <vilib>:"Mean.vi"("X"=w545) -> ("mean"=w544:dbl)  [unwired: 1 out]
          n198 = call "Read_value_of_earlier_Ch.vi"("Desired Ch to Read"=w534, "Ch names"=w535, "Present scan array"=w536) -> ("Value"=w526:dbl)  [unwired: 1 in, 1 out]
          n199 = Not Equal?(x=w526, y=w525) -> (x != y?=w524:bool)
          n200 = Max & Min(x=w526, y=w525) -> (min(x,y)=w527:dbl)  [unwired: 1 out]
          n201 = Greater?(x=w544, y=w537) -> (0:w532:bool)
          n202 = Less?(x=w527, y=7.0) -> (x < y?=w531:bool)
          n203 = Compound Arithmetic op=OR(w532, w531, w524) -> (w530:bool)
          n204 = case shown="False" w530 {
            tunnel: w543 -> [w565 w570]
            tunnel: [w557 w570] -> w542
            tunnel: w541 -> [w564 _]
            tunnel: w540 -> [w568 _]
            tunnel: w536 -> [w567 _]
            tunnel: w535 -> [w566 _]
            tunnel: w539 -> [w563 w569]
            tunnel: [w552 w569] -> w538
            tunnel: w526 -> [w546 _]
            frame False {
              # "Setpoint"
              # "Current"
              n205 = call "Read_value_of_earlier_Ch.vi"("Desired Ch to Read"=w568, "Ch names"=w566, "Present scan array"=w567) -> ("Value"=w562:dbl)  [unwired: 1 in, 1 out]
              n206 = Format Into String(format string="%s has a setpoint temp of %.1f and a measured temp of %.1f.\n", initial string=w565, w564, w546, w562) -> (resulting string=w558:string)  [unwired: 1 in, 1 out]
              n207 = Subtract(x=w546, y=w562) -> (x-y=w561:dbl)
              n208 = Format Into String(format string="%s has a setpoint temp of %.1f and a measured temp of %d.\n", initial string=w563, w564, w546, w562) -> (resulting string=w555:string)  [unwired: 1 in, 1 out]
              n209 = Greater?(x=w546, y=0.02) -> (0:w548:bool)
              n210 = Absolute Value(x=w561) -> (abs(x)=w560:dbl)
              n211 = Greater?(x=w560, y=0.2) -> (0:w549:bool)
              n212 = And(x=w549, y=w548) -> (x .and. y?=w547:bool)
              n213 = Select(t=w558, s=w547, f="") -> (s? t:f=w557:string)
              n214 = Select(t=w555, s=w547, f="") -> (s? t:f=w552:string)
            }
            frame True {
            }
          }
        }
        n215 = Select(t=w499, s=w500, f="") -> (s? t:f=w497:string)
        n216 = while {
          tunnel: w505 -> [w515]
          shift-right: [w512] -> _
          shift-left: _ -> [w513]
          tunnel: w497 -> [w512]
          stop <- TRUE stop-if-true
          n217 = Not Equal?(x=w512, y=w513) -> (x != y?=w517:bool)
          n218 = Empty String/Path?(string/path=w512) -> (empty?=w516:bool)
          n219 = Compound Arithmetic op=AND(w517, invert w516) -> (w514:bool)
          n220 = case shown="True" w514 {
            tunnel: w515 -> [_ w520]
            frame False {
            }
            frame True {
              n221 = Format Into String(format string="The following channels have currently have a zero power demand:\n\n%s\n\n \nPlease check that this is not adversly affecting your experimental conditions.", w520) -> (resulting string=w519:string)  [unwired: 2 in, 1 out]
              n222 = call "Server_Emails.vi"("Client Name Contains"="EnFlo_Tunnel", "Message"=w519, "Subject"="Zero Heater Power Warning" ("t")) -> ()  [unwired: 2 in, 3 out]
            }
          }
        }
      }
      frame #7 {
        n223 = case shown="True" w571 {
          frame False {
          }
          frame True {
            n224 = Build Array("EnFlo_Tunnel:Heater:Enable") -> (w574:string[])
            n225 = Build Array(0.0) -> (w572:dbl[])
            n226 = call "ASYNC_Adam_server.vi"("Values"=w572, "Channel Names"=w574) -> ()  [unwired: 1 in, 3 out]
          }
        }
      }
    }
  }
